vi "From PV Data.vi"(8 "error in":errorcluster, 10 "PV data in":refnum<class "PV Data.lvclass">, 11 "Base Interface in":refnum<class "Base Interface.lvclass">) -> (0 "error out":errorcluster, 2 "PV data out":refnum<class "PV Data.lvclass">, 3 "Base Interface out":refnum<class "Base Interface.lvclass">)   [LabVIEW 2020, in "PV Access.lvlib" / "PV Data.lvlib" / "Base Interface.lvclass"]
uses:
  Base Interface.lvclass
  PV Data/PV Data.lvclass
  PV Data/Read Field - Variant.vi
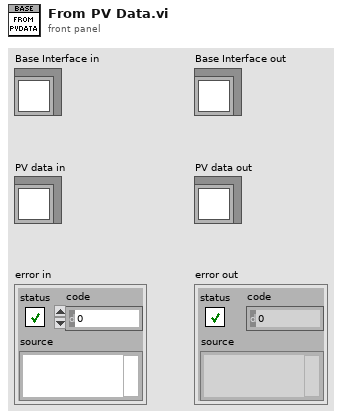
[diagram p1: front panel]
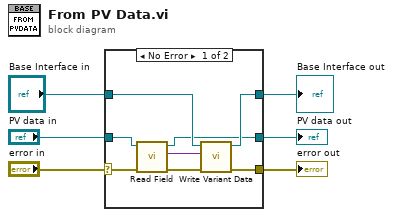
[diagram p0: block diagram]
diagram:
  n1 = case shown="No Error" "error in" {
    selector: "error in" -> [w12 w17]
    tunnel: [w11 w17] -> w1
    tunnel: [w10 w16] -> w3
    tunnel: "Base Interface in" -> [w9 w16]
    tunnel: "PV data in" -> [w8 w15]
    tunnel: [w7 w15] -> w2
    frame No Error {
      n2 = call-poly "Read Field.vi"("error in (no error)"=w12, "PV Data in"=w8) -> ("error out"=w14:errorcluster, "value out"=w13:variant, "PV Data out"=w7:refnum<class "PV Data.lvclass">)  [unwired: 6 in, 1 out]
      n3 = call-dynamic "Write Variant Data.vi"("error in (no error)"=w14, "data"=w13, "Base Interface in"=w9) -> ("error out"=w11:errorcluster, "Base Interface out"=w10:refnum<class "Base Interface.lvclass">)  [unwired: 7 in]
    }
    frame Error {
    }
  }
  "error out" <- w1
  "Base Interface out" <- w3
  "PV data out" <- w2
